vi "Post-Build Action.vi"(5 "Files Generated by Build":path[](array[path]), 6 "Top Level/Always Included VIs":path[](array[path]), 7 "Destination Path":path, 8 "error in (no error)":errorcluster, 9 "Target Name":string, 10 "Build Specification Name":string, 11 "Project Path":path) -> (0 "error out":errorcluster)   [LabVIEW 2020]
uses:
  <vilib>/Utility/lvfile.llb/NI_FileType.lvlib
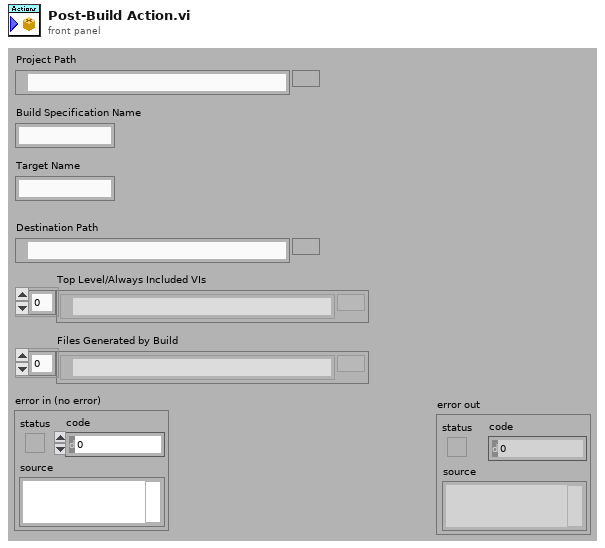
[diagram p1: front panel]
types:
  T1 = typedef "NI_FileType.lvlib/FT_FileTypes.ctl" = enum32{"Invalid file/path", "Unknown type", "Instrument", "Control", "Polymorphic VI", "Project", "Library", "LVClass", "XControl", "XNode", "CIN", "Run-time menu", "Palette menu", "LLB", "Shortcut", "Directory", "Class Private Data Control", "Statechart", "MathScript .m file", "Ladder Diagram", "LVLibp"}
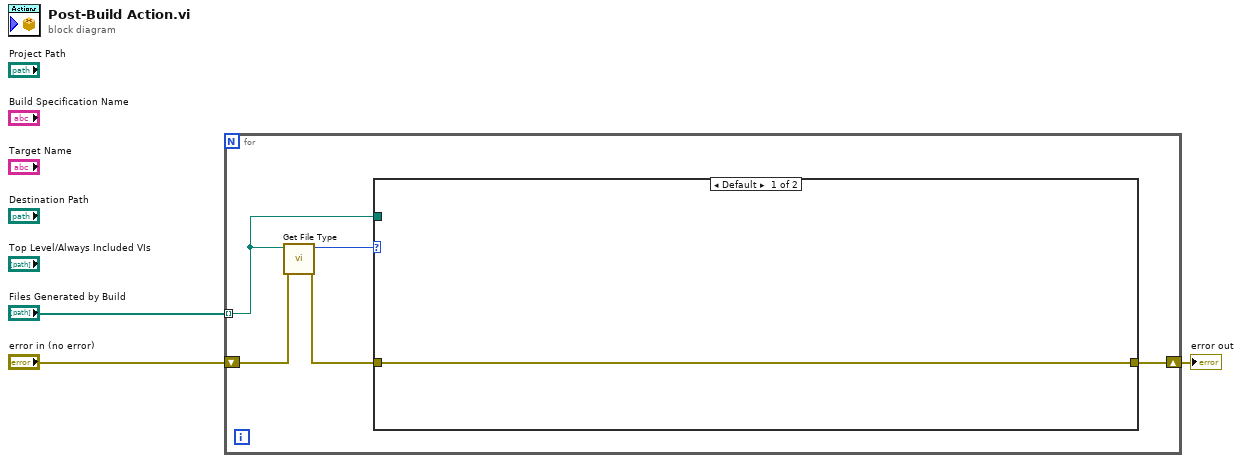
[diagram p0: block diagram]
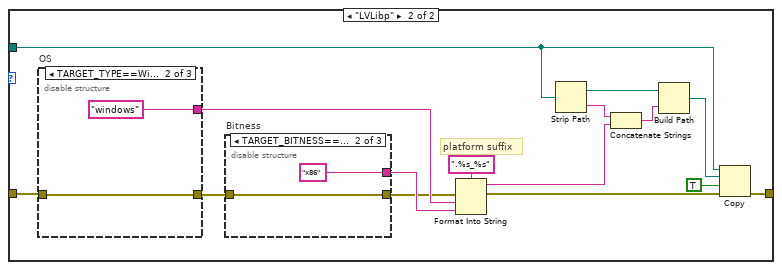
[diagram p2: hidden frame]
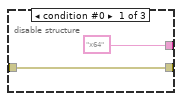
[diagram p3: hidden frame]
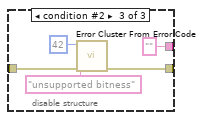
[diagram p4: hidden frame]
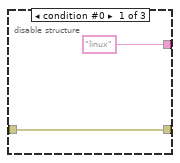
[diagram p5: hidden frame]
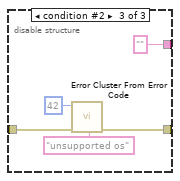
[diagram p6: hidden frame]
diagram:
  n1 = for {
    shift-right: [w8] -> w2
    shift-left: "error in (no error)" -> [w7]
    tunnel: "Files Generated by Build" -> [w5] mode=indexing
    n2 = call <vilib>:"Get File Type.vi"("error in (no error)"=w7, "path"=w5) -> ("error out"=w6:errorcluster, "file type"=w4:T1)  [unwired: 7 in, 1 out]
    n3 = case shown="Default" w4 {
      tunnel: w6 -> [w9 w19]
      tunnel: [w9 w14] -> w8
      tunnel: w5 -> [_ w10]
      frame Default {
      }
      frame "LVLibp" {
        # "platform suffix"
        n4 = disable-structure "OS" shown="TARGET_TYPE==Windows" {
          disable-tunnel: ["linux" "windows" ""] -> w23
          disable-tunnel: [w34 w36 w39] -> w24
          disable-tunnel: w19 -> [w34 w36 w38]
          frame condition #0 {
          }
          frame condition #1 (active) {
          }
          frame condition #2 {
            n5 = call <vilib>:"Error Cluster From Error Code.vi"("error in (no error)"=w38, "error message (\"\")"="unsupported os" ("error message (\"\")"), "error code (0)"=42) -> ("error out"=w39:errorcluster)  [unwired: 6 in]
          }
        }
        n6 = disable-structure "Bitness" shown="TARGET_BITNESS==32" {
          disable-tunnel: ["x64" "x86" ""] -> w22
          disable-tunnel: w24 -> [w25 w27 w30]
          disable-tunnel: [w25 w27 w29] -> w20
          frame condition #0 {
          }
          frame condition #1 (active) {
          }
          frame condition #2 {
            n7 = call <vilib>:"Error Cluster From Error Code.vi"("error in (no error)"=w30, "error message (\"\")"="unsupported bitness" ("error message (\"\")"), "error code (0)"=42) -> ("error out"=w29:errorcluster)  [unwired: 6 in]
          }
        }
        n8 = Format Into String(format string=".%s_%s", error in=w20, w23, w22) -> (resulting string=w17:string, error out=w12:errorcluster)  [unwired: 1 in]
        n9 = Strip Path(path=w10) -> (stripped path=w15:path, name=w18:string)
        n10 = Concatenate Strings(w18, w17) -> (w16:string)
        n11 = Build Path(base path=w15, name or relative path=w16) -> (appended path=w13:path)
        n12 = Copy(8:w12, 9:TRUE ("overwrite (F)"), 10:w13, 11:w10) -> (0:w14:errorcluster)  [unwired: 1 in, 2 out]
      }
    }
  }
  "error out" <- w2
